vi "Emballage_BDD_chargement_Code_Barre_Fixe_fin.vi"(8 "Error in":errorcluster caption="Error in (no error)", 11 "code_barre_fixe_fin":string) -> (0 "Error out":errorcluster, 2 "code_barre_fixe_fichier?":bool, 3 "tbl_Autre_Article":string[][](array[string]))   [LabVIEW 2020]
uses:
  <vilib>/Utility/file.llb/Read Delimited Spreadsheet (string).vi
panel:
  out "champ":string
  out "Chemin":string
  out "tableau sans le sous-tableau":string[][](array[string])
  out "indice de l'élément \"index\"":i32
  out "indice de l'élément \"Autre\"":i32
  out "first row":string[](array[string]) caption="première ligne"
  out "all rows":string[][](array[string]) caption="toutes les lignes"
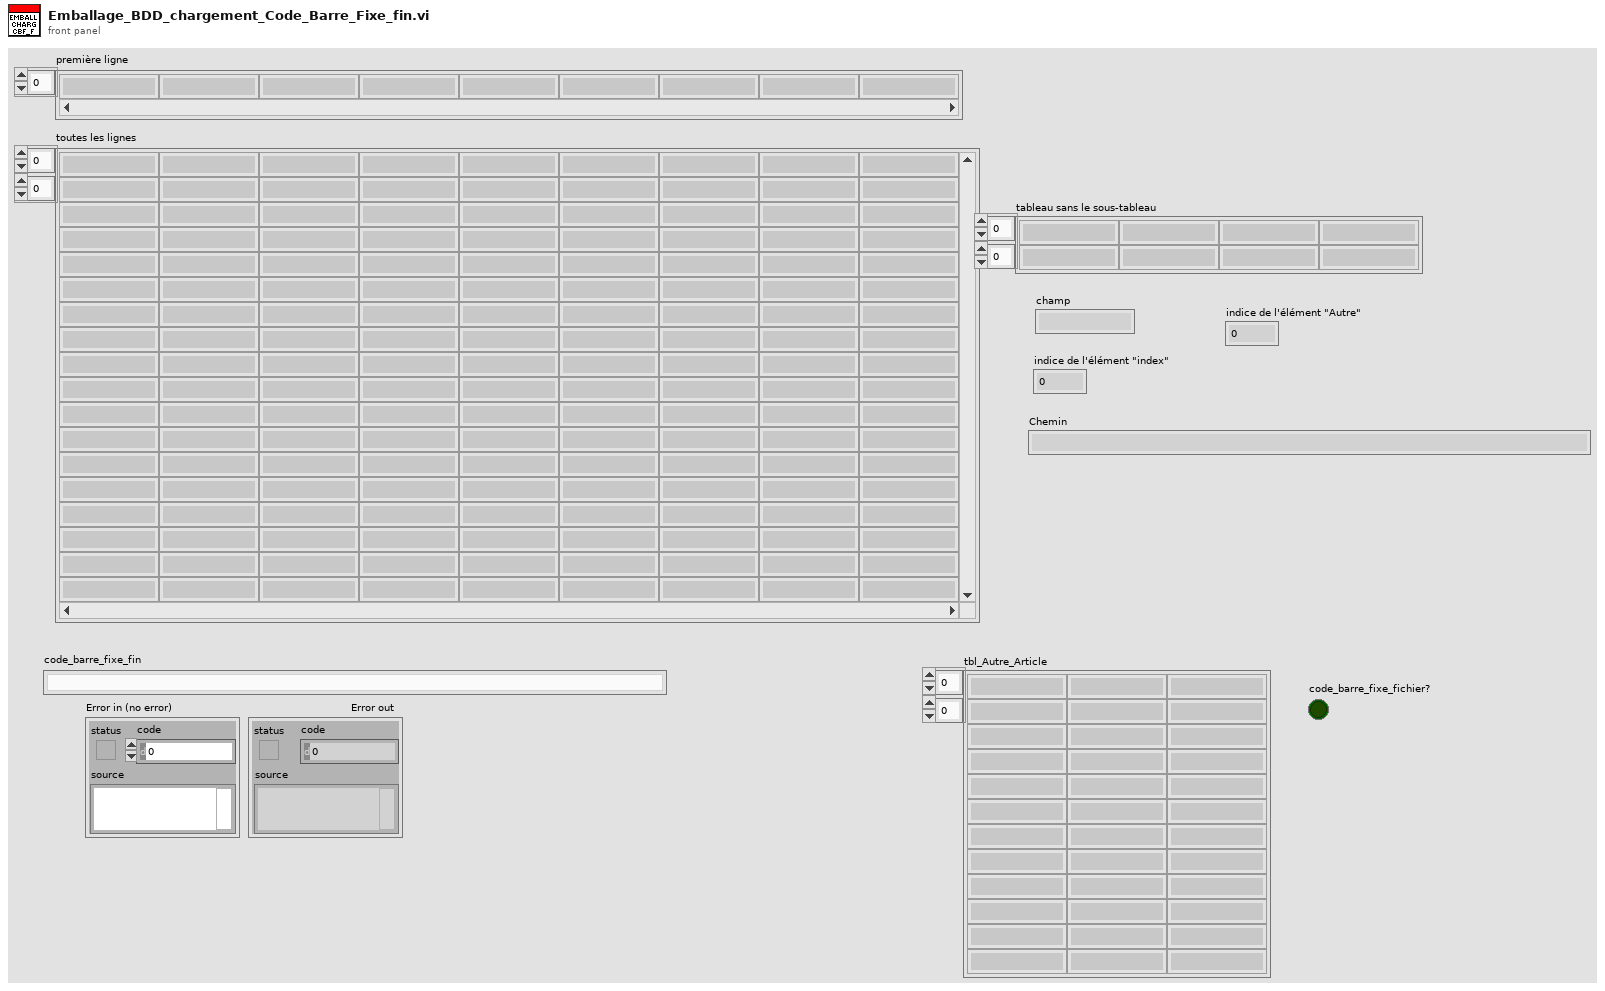
[diagram p1: front panel]
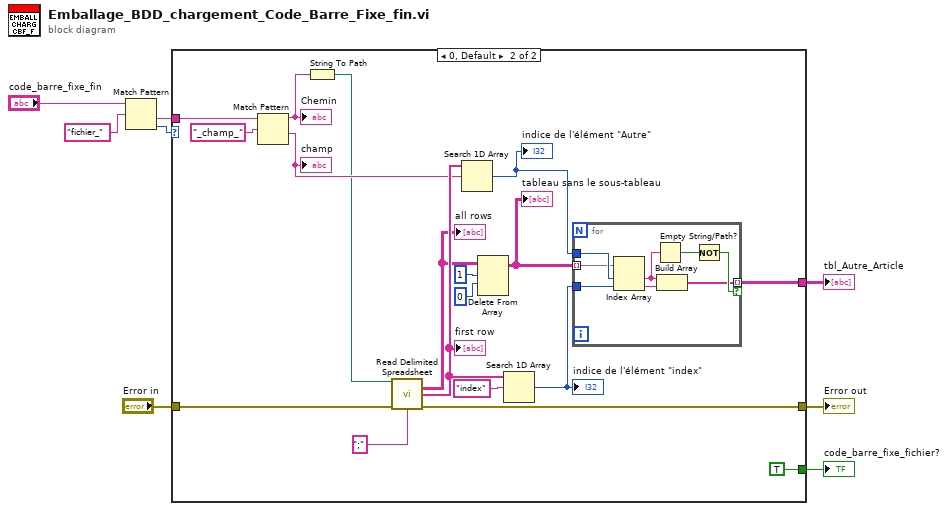
[diagram p0: block diagram]
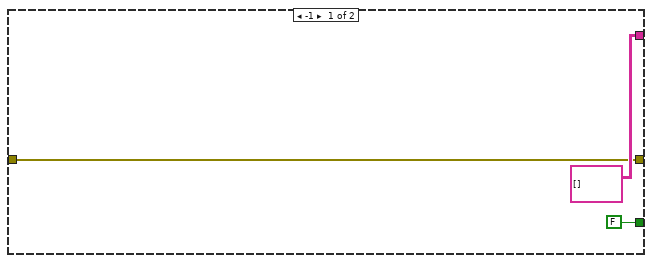
[diagram p2: hidden frame]
diagram:
  n1 = Match Pattern(string="code_barre_fixe_fin", regular expression="fichier_" ("expression régulière")) -> (after substring=w6:string, offset past match=w5:i32)  [unwired: 1 in, 2 out]
  n2 = case shown="0, Default" w5 {
    tunnel: w6 -> [_ w21]
    tunnel: [string[][] [] w15] -> w4
    tunnel: [FALSE TRUE] -> w3
    tunnel: "Error in" -> [w9 w13]
    tunnel: [w9 w12] -> w1
    frame -1 {
    }
    frame 0, Default {
      n3 = Match Pattern(string=w21, regular expression="_champ_" ("expression régulière")) -> (before substring=w18:string, after substring=w19:string)  [unwired: 1 in, 2 out]
      "Chemin" <- w18
      "champ" <- w19
      n4 = String To Path(string=w18) -> (path=w17:path)
      n5 = call-poly <vilib>:"Read Delimited Spreadsheet.vi"("file path (dialog if empty)"=w17, "error in (no error)"=w13, "delimiter (\\t)"=";" ("delimiter (\\t)")) -> ("all rows"=w26:string[][], "first row"=w27:string[], "error out"=w12:errorcluster)  [unwired: 7 in, 3 out]
      "all rows" <- w26
      "first row" <- w27
      n6 = Search 1D Array(1D array=w27, element=w19) -> (index of element=w22:i32)  [unwired: 1 in]
      "indice de l'élément \"Autre\"" <- w22
      n7 = Delete From Array(array=w26, length=1 ("longueur"), index (row)=0 ("indice (ligne)")) -> (array with subset deleted=w23:string[][])  [unwired: 1 in, 1 out]
      "tableau sans le sous-tableau" <- w23
      n8 = Search 1D Array(1D array=w27, element="index" ("élément")) -> (index of element=w16:i32)  [unwired: 1 in]
      "indice de l'élément \"index\"" <- w16
      n9 = for {
        tunnel: w23 -> [w34] mode=indexing
        tunnel: w22 -> [w37]
        tunnel: [w33] -> w15 mode=indexing if=w35
        tunnel: w16 -> [w30]
        n10 = Index Array(array=w34, index #1=w37, index #2=w30) -> (element #1=w32:string, element #2=w31:string)
        n11 = Empty String/Path?(string/path=w32) -> (empty?=w36:bool)
        n12 = Build Array(w32, w31) -> (w33:string[])
        n13 = Not(x=w36) -> (.not. x?=w35:bool)
      }
    }
  }
  "tbl_Autre_Article" <- w4
  "code_barre_fixe_fichier?" <- w3
  "Error out" <- w1
